vi "GetType.vi"(8 "error in (no error)":errorcluster, 11 "Abort Generation Msg":refnum<class "Abort Generation Msg.lvclass">) -> (0 "error out":errorcluster, 2 "Data Sample":variant, 3 "Abort Generation Msg":refnum<class "Abort Generation Msg.lvclass">)   [LabVIEW 2015, in "CS++Fgen.lvlib" / "Abort Generation Msg.lvclass"]
doc: "This VI delivers a sample of the data type format the message expects."
uses:
  Abort Generation Msg.lvclass
  Abort Generation Msg.lvclass/Abort Generation Msg.ctl
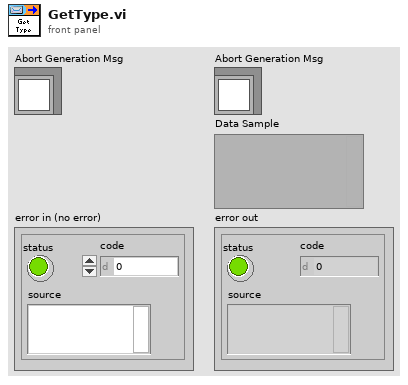
[diagram p1: front panel]
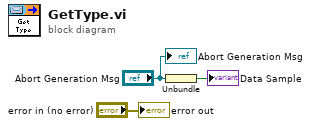
[diagram p0: block diagram]
diagram:
  n1 = Unbundle("Abort Generation Msg") -> (→"Data Sample":bool)
  "error out" <- "error in (no error)"
  "Abort Generation Msg" <- "Abort Generation Msg"
